vi "Set Prefix.vi"(8 "error in (no error)":errorcluster, 10 "Prefix":string, 11 "ExperimentService in":refnum<class "ExperimentService.lvclass">) -> (0 "error out":errorcluster, 3 "ExperimentService out":refnum<class "ExperimentService.lvclass">)   [LabVIEW 2014, in "ExperimentService.lvclass"]
uses:
  ExperimentService.lvclass
  <vilib>/ActorFramework/Message Enqueuer/Message Priority.ctl
  ExperimentService.lvclass/ExperimentService.ctl
  StorageService/StorageService Messages/Write Prefix Msg/Write Prefix Msg.lvclass/Write Prefix Msg.ctl
  <vilib>/ActorFramework/Message Enqueuer/Message Enqueuer.lvclass/Message Enqueuer.ctl
  <vilib>/ActorFramework/Message Enqueuer/Enqueue.vi
  <vilib>/ActorFramework/Message Priority Queue/Priority Enqueue.vi
  StorageService/StorageService Messages/Write Prefix Msg/Write Prefix Msg.lvclass
  <vilib>/ActorFramework/Message Enqueuer/Message Enqueuer.lvclass
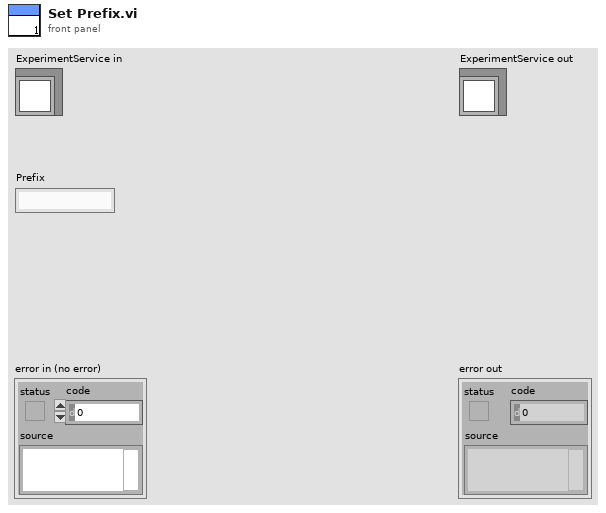
[diagram p1: front panel]
types:
  T1 = typedef "Actor Framework.lvlib/Message Enqueuer.lvclass/Message Priority.ctl" = enum16{"Low", "Normal", "High"}
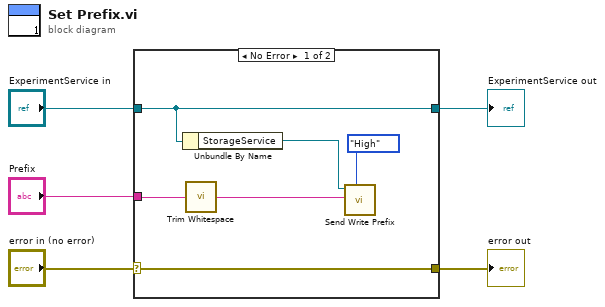
[diagram p0: block diagram]
diagram:
  n1 = case shown="No Error" "error in (no error)" {
    selector: "error in (no error)" -> [w11 w13]
    tunnel: [w11 w13] -> w4
    tunnel: [w10 w12] -> w2
    tunnel: "ExperimentService in" -> [w10 w12]
    tunnel: "Prefix" -> [w7 _]
    frame No Error {
      n2 = Unbundle By Name(w10) -> ("StorageService"=w9:refnum<class "Message Enqueuer.lvclass">)
      n3 = call <vilib>:"Trim Whitespace.vi"("string"=w7) -> ("trimmed string"=w6:string)  [unwired: 1 in]
      n4 = call "Send Write Prefix.vi"("Message Priority (Normal)"=Message_Priority."High", "Prefix"=w6, "Message Enqueuer"=w9) -> ()  [unwired: 7 in, 2 out]
    }
    frame Error {
    }
  }
  "error out" <- w4
  "ExperimentService out" <- w2
